vi "UtilityLib.merge errors.vi"(1 "error2 (no error)":errorcluster, 2 "error1 (no error)":errorcluster) -> (0 "error out":errorcluster)   [LabVIEW 2014, in "UtilityLib.lvlib"]
doc: "Merges two errors in the following way:\n\n\"error1\" and \"error2\" have same priority: \"error1\" is returned\n\"error1\" and \"error2\" have different priority: the \"errorx\" with higher priority is returned.\n\nThis error merge is optimized for speed."
uses:
  UtilityLib.lvlib
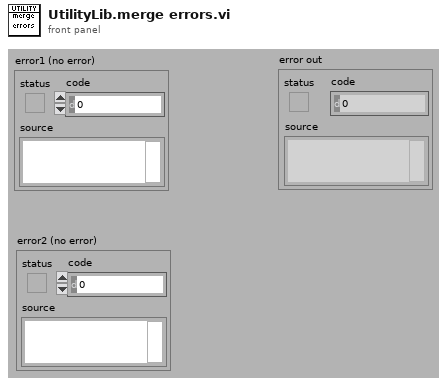
[diagram p1: front panel]
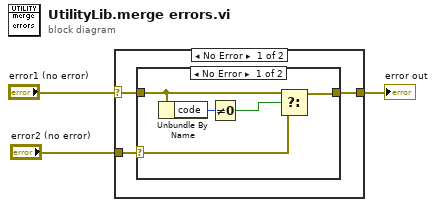
[diagram p0: block diagram]
diagram:
  n1 = case shown="No Error" "error1 (no error)" {
    selector: "error1 (no error)" -> [w4 w13]
    tunnel: [w5 w13] -> w2
    tunnel: "error2 (no error)" -> [w6 _]
    frame No Error {
      n2 = case shown="No Error" w6 {
        selector: w6 -> [w8 w12]
        tunnel: [w7 w12] -> w5
        tunnel: w4 -> [w9 _]
        frame No Error {
          n3 = Unbundle By Name(w9) -> ("code"=w11:i32)
          n4 = Not Equal To 0?(x=w11) -> (x != 0?=w10:bool)
          n5 = Select(t=w9, s=w10, f=w8) -> (s? t:f=w7:errorcluster)
        }
        frame Error {
        }
      }
    }
    frame Error {
    }
  }
  "error out" <- w2
